vi "Create.vi"(6 "timeout (-1)":i32=-1, 7 "EventDaemon in":refnum<class "ErrorHandler.lvclass">, 8 "error in (no error)":errorcluster) -> (0 "error out":errorcluster, 3 "EventDaemon out":refnum<class "ErrorHandler.lvclass">)   [LabVIEW 2024, in "ErrorHandler.lvclass"]
doc: "Creates daemon class. By default, timeout is -1 and will wait for event messages. Set to millisecond delay time if a specific cycle time is required"
uses:
  ErrorHandler.lvclass
  ErrorHandler.lvclass/ErrorHandler.ctl
  states--enum.ctl
  status--cluster.ctl
  msg--cluster.ctl
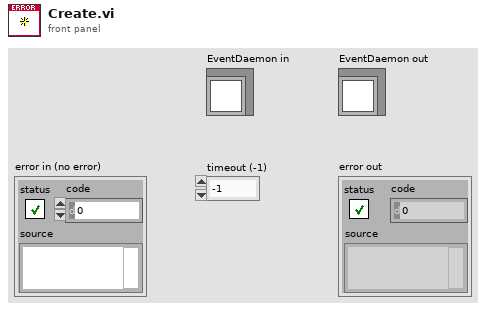
[diagram p1: front panel]
types:
  T1 = typedef "ErrorHandler.lvclass/states--enum.ctl" = enum16{"init", "default", "display error", "error handler", "exit"}
  T2 = typedef "ErrorHandler.lvclass/msg--cluster.ctl" = cluster{"cmd":T1, "error":errorcluster}
  T3 = typedef "ErrorHandler.lvclass/status--cluster.ctl" = cluster{"loop time":u32, "current state":T1, "error":errorcluster}
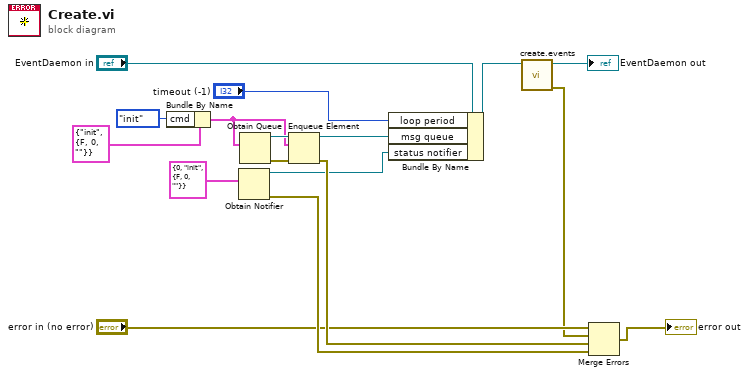
[diagram p0: block diagram]
diagram:
  n1 = Bundle By Name(cluster=T2 {"cmd"=enum."init", "error"={"status"=FALSE, "code"=0, "source"=""}} ("msg"), "cmd"=states--enum."init") -> (w2:T2)
  n2 = Obtain Notifier(notification data type=T3 {"loop time"=0, "current state"=enum."init", "error"={"status"=FALSE, "code"=0, "source"=""}} ("status")) -> (notifier out=w8:refnum<notifier>, error out=w7:errorcluster)  [unwired: 3 in, 1 out]
  n3 = Obtain Queue(element data type=w2) -> (queue out=w12:refnum<queue>, error out=w11:errorcluster)  [unwired: 4 in, 1 out]
  n4 = Enqueue Element(queue=w12, element=w2, error in (no error)=w11) -> (queue out=w1:refnum<queue>, error out=w10:errorcluster)  [unwired: 1 in, 1 out]
  n5 = Bundle By Name(cluster="EventDaemon in", "loop period"="timeout (-1)", "msg queue"=w1, "status notifier"=w8) -> (w14:refnum<class "ErrorHandler.lvclass">)
  n6 = call "create.events.vi"("EventDaemon in"=w14) -> ("error out"=w5:errorcluster, "EventDaemon out"=→"EventDaemon out":refnum<class "ErrorHandler.lvclass">)  [unwired: 9 in]
  n7 = Merge Errors("error in (no error)", w5, w10, w7) -> (→"error out":errorcluster)
